vi "COMI DO Get All.vi"(11 "hDevice":u32) -> (2 "function return":u32, 3 "hDevice out":u32)   [LabVIEW 2017, in "Comidll.lvlib"]
doc: "unsigned long (COMI_DO_GetAll) (HANDLE hDevice);"
uses:
  <userlib>/Comidll/Comidll.lvlib
  <userlib>/Comidll/Comidll.dll
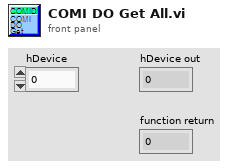
[diagram p1: front panel]
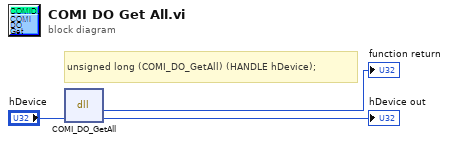
[diagram p0: block diagram]
diagram:
  # "unsigned long\t(COMI_DO_GetAll) (HANDLE hDevice);"
  n1 = dll-call lib="C:/Program Files/National Instruments/LabVIEW 2017/user.lib/Comidll/Comidll.*" fn="COMI_DO_GetAll"("hDevice"="hDevice") -> (→"function return":u32, "hDevice"=→"hDevice out":u32)  [unwired: 3 in, 2 out]
